vi "CryptoNight-Step-3.vi"(9 "Override Iterations":bool=TRUE, 10 "# of Iterations":i32, 11 "FileName":string="log_file.8.bin") -> (1 "hp_state out":u8[](array[numeric]) format="%.0x", 2 "b_out":u64[](array[numeric]) format="%.0x", 3 "a_out":u64[](array[numeric]) format="%.0x")   [LabVIEW 2017]
uses:
  MixColumn.vi
  Convert-U32-U8-Array.vi
  xtime.vi
  Create S box Number.vi
  Shift Rows.vi
  Add Roundkey.vi
panel:
  out "appended array":u8[](array[numeric]) format="%.0x"
  out "j2":i32
  out "j":u64
  out "i":i32
  out "# of Iterations":i32
  in  "error in":errorcluster
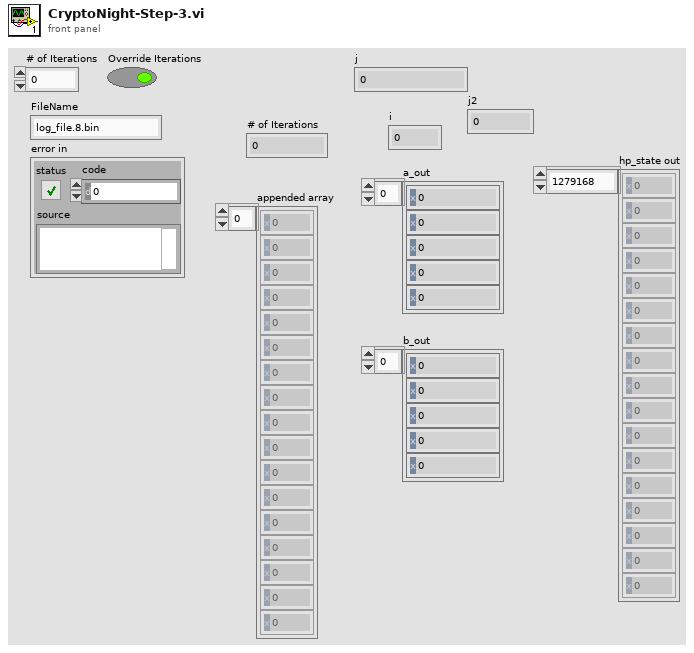
[diagram p1: front panel]
types:
  T1 = cluster{"a":u64[], "b":u64[], "hp_state_in":u8[], "hp_state_out":u8[]}
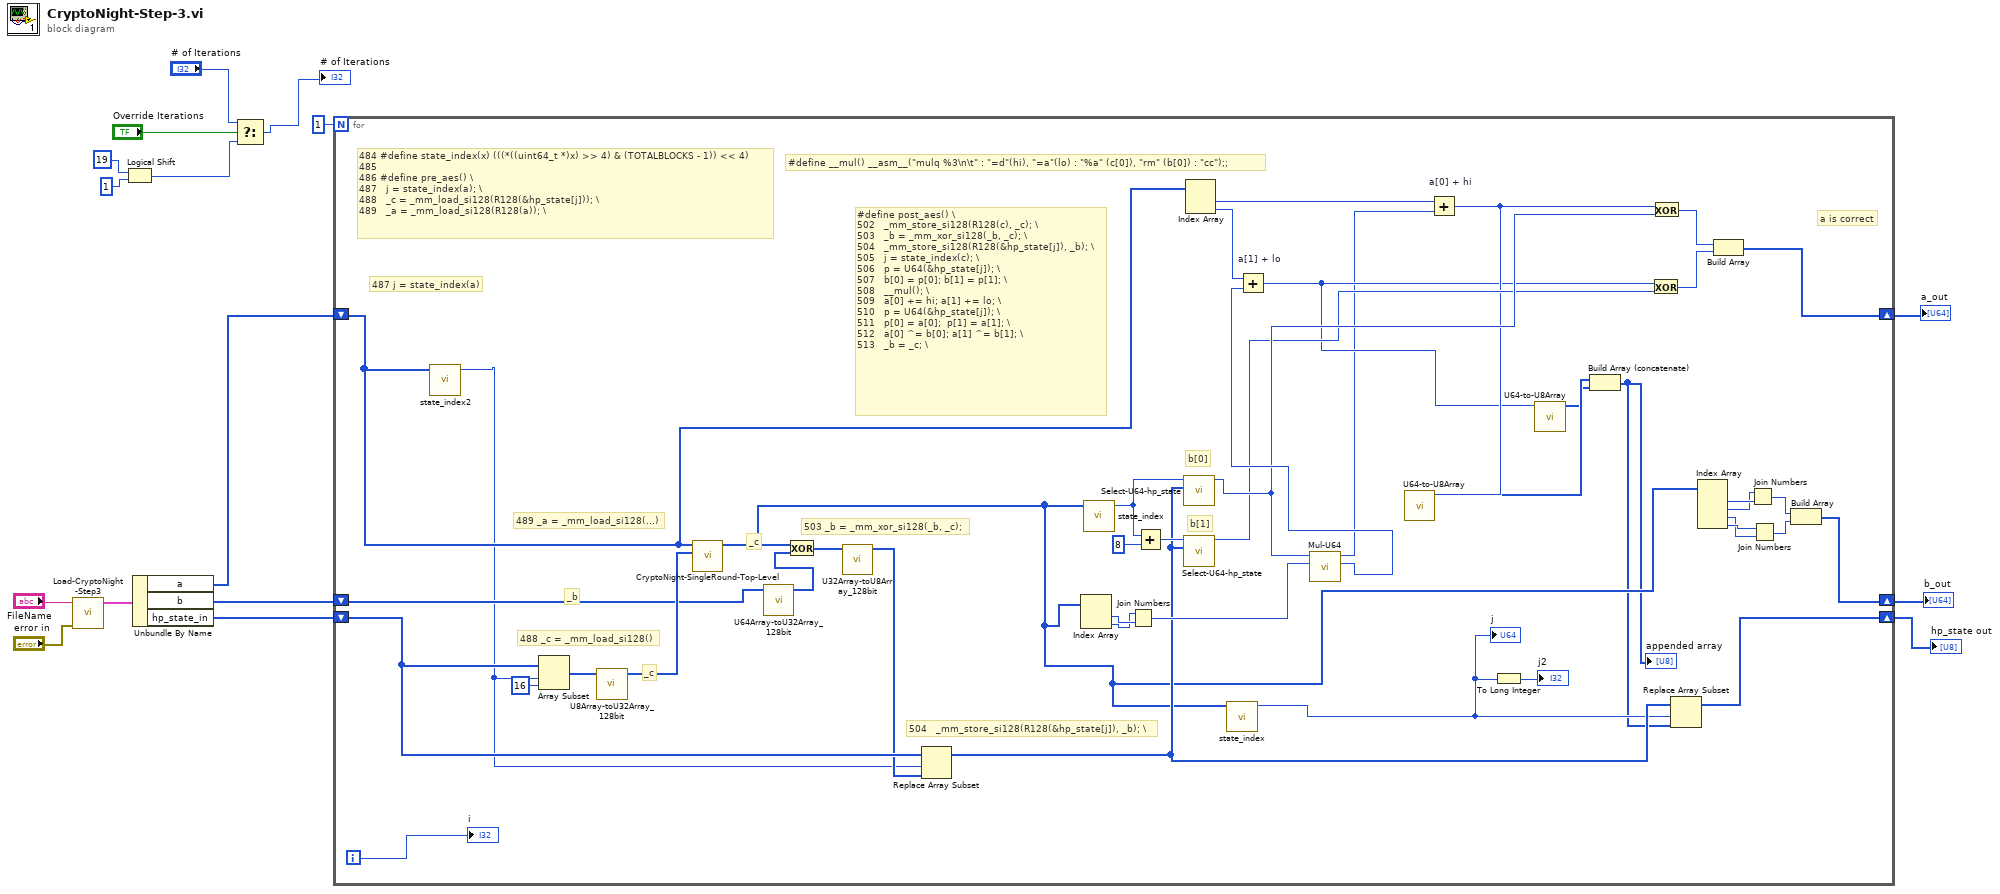
[diagram p0: block diagram]
diagram:
  n1 = call "Load-CryptoNight-Step3.vi"("error in"="error in", "FileName"="FileName") -> ("output cluster"=w12:T1)  [unwired: 8 in, 1 out]
  n2 = Logical Shift(y=19, x=1) -> (x << y=w4:i32)
  n3 = Unbundle By Name(w12) -> ("a"=w10:u64[], "b"=w9:u64[], "hp_state_in"=w11:u8[])
  n4 = Select(t="# of Iterations", s="Override Iterations", f=w4) -> (s? t:f=→"# of Iterations":i32)
  n5 = for {
    N: 1 -> [_]
    shift-right: [w23] -> w8
    shift-left: w9 -> [w33]
    shift-right: [w46] -> w6
    shift-left: w11 -> [w56]
    shift-right: [w40] -> w7
    shift-left: w10 -> [w18]
    i -> [w22]
    # "a is correct"
    # "b[1]"
    # "b[0]"
    # "#define __mul() __asm__(\"mulq %3\\n\\t\" : \"=d\"(hi), \"=a\"(lo) : \"%a\" (c[0]), \"rm\" (b[0]) : \"cc\");;"
    # "489 _a = _mm_load_si128(...)"
    # "_c"
    # "_c"
    # "_b"
    # "504   _mm_store_si128(R128(&hp_state[j]), _b); \\"
    # "503 _b = _mm_xor_si128(_b, _c);"
    # "488 _c = _mm_load_si128()"
    # "487 j = state_index(a)"
    # "#define post_aes() \\\n502   _mm_store_si128(R128(c), _c); \\\n503   _b = _mm_xor_si128(_b, _c); \\\n504   _mm_store_si128(R128(&hp_state[j]), _b); \\\n505   j = state_index(c); \\\n506   p = U64(&hp_state[j]); \\\n507   b[0] = p[0]; b[1] = p[1]; \\\n508   __mul(); \\\n509   a[0] += hi; a[1] += lo; \\\n510   p = U64(&hp_state[j]); \\\n511   p[0] = a[0];  p[1] = a[1]; \\\n512   a[0] ^= b[0]; a[1] ^= b[1]; \\\n513   _b = _c; \\"
    # "484 #define state_index(x) (((*((uint64_t *)x) >> 4) & (TOTALBLOCKS - 1)) << 4)\n485 \n486 #define pre_aes() \\\n487   j = state_index(a); \\\n488   _c = _mm_load_si128(R128(&hp_state[j])); \\\n489   _a = _mm_load_si128(R128(a)); \\"
    n6 = call "state_index2.vi"("2 x U64"=w18) -> ("j"=w17:u64)  [unwired: 10 in]
    n7 = Array Subset(array=w56, index=w17, length=16) -> (w58:u8[])
    n8 = call "U8Array-toU32Array_128bit.vi"("16 x U8"=w58) -> ("4 x U32"=w57:u32[])  [unwired: 10 in]
    n9 = call "CryptoNight-SingleRound-Top-Level.vi"("state (c)"=w57, "key (a)"=w18) -> ("state out (c)"=w25:u32[])  [unwired: 9 in]
    n10 = call "U64Array-toU32Array_128bit.vi"("2 x U64"=w33) -> ("4 x U32"=w32:u32[])  [unwired: 10 in]
    n11 = Exclusive Or(1:w32, 2:w25) -> (0:w55:u32[])
    n12 = call "U32Array-toU8Array_128bit.vi"("4 x U32"=w55) -> ("16 x U8"=w54:u8[])  [unwired: 10 in]
    n13 = Replace Array Subset(array=w56, new element=w54, index=w17) -> (w47:u8[])
    n14 = Index Array(array=w25) -> (element #1=w50:u32, element #2=w49:u32)  [unwired: 2 in]
    n15 = call "state_index.vi"("4 x U32 2"=w25) -> ("j"=w52:u64)  [unwired: 10 in]
    n16 = Join Numbers(hi=w49, lo=w50) -> ((hi.lo)=w48:u64)
    n17 = Add(x=w52, y=u64 8 ("x")) -> (x+y=w53:u64)
    n18 = call "Select-U64-hp_state.vi"("hp_state_in"=w47, "j"=w52) -> ("U64(hp_state[j])"=w42:u64)  [unwired: 9 in]
    n19 = call "Select-U64-hp_state.vi"("hp_state_in"=w47, "j"=w53) -> ("U64(hp_state[j])"=w41:u64)  [unwired: 9 in]
    n20 = Index Array(array=w18) -> (element #1=w45:u64, element #2=w44:u64)  [unwired: 2 in]
    n21 = call "state_index.vi"("4 x U32 2"=w25) -> ("j"=w21:u64)  [unwired: 10 in]
    "j" <- w21
    n22 = call "Mul-U64.vi"("c[0]"=w48, "b[0]"=w42) -> ("lo"=w43:u64, "hi"=w24:u64)  [unwired: 8 in]
    n23 = Add "a[1] + lo"(x=w44, y=w43) -> (x+y=w34:u64)
    n24 = Add "a[0] + hi"(x=w45, y=w24) -> (x+y=w37:u64)
    n25 = call "U64-to-U8Array.vi"("Numeric"=w37) -> ("Array"=w36:u8[])  [unwired: 10 in]
    n26 = To Long Integer(number=w21) -> (32bit integer=→"j2":i32)
    n27 = call "U64-to-U8Array.vi"("Numeric"=w34) -> ("Array"=w35:u8[])  [unwired: 10 in]
    n28 = Build Array (concatenate)(w36, w35) -> (w19:u8[])
    "appended array" <- w19
    n29 = Exclusive Or(1:w41, 2:w34) -> (0:w38:u64)
    n30 = Exclusive Or(1:w42, 2:w37) -> (0:w39:u64)
    n31 = Replace Array Subset(array=w47, new element=w19, index=w21) -> (w46:u8[])
    n32 = Index Array(array=w25) -> (element #1=w31:u32, element #2=w30:u32, element #3=w28:u32, element #4=w29:u32)  [unwired: 4 in]
    n33 = Build Array(w39, w38) -> (w40:u64[])
    n34 = Join Numbers(hi=w30, lo=w31) -> ((hi.lo)=w27:u64)
    n35 = Join Numbers(hi=w29, lo=w28) -> ((hi.lo)=w26:u64)
    n36 = Build Array(w27, w26) -> (w23:u64[])
    "i" <- w22
  }
  "b_out" <- w8
  "a_out" <- w7
  "hp_state out" <- w6
